vi "Dispose.vi"(8 "error in (no error)":errorcluster, 11 "ProductA":refnum<class "ProductA.lvclass">) -> (0 "error out":errorcluster)   [LabVIEW 2020, in "FactoryMethod.lvlib" / "FactoryMethodLazyEvaluation.lvlib" / "ProductA.lvclass"]
uses:
  ProductA.lvclass
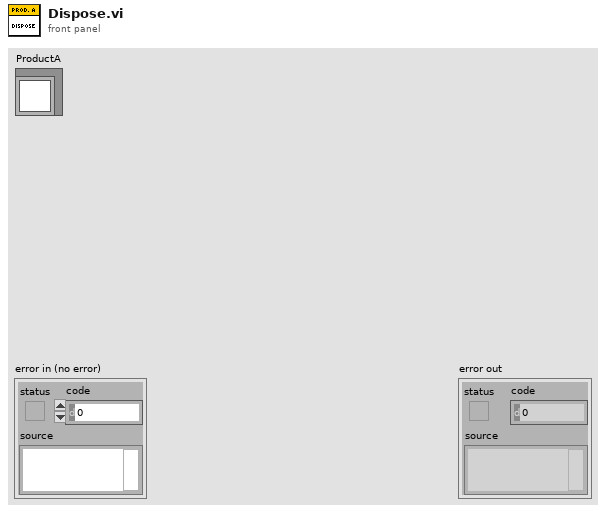
[diagram p1: front panel]
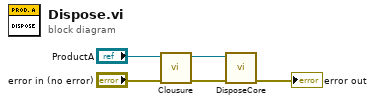
[diagram p0: block diagram]
diagram:
  n1 = call-dynamic "Clousure.vi"("error in (no error)"="error in (no error)", "ProductA"="ProductA") -> ("error out"=w3:errorcluster, "ProductA"=w1:refnum<class "ProductA.lvclass">)  [unwired: 8 in]
  n2 = call-dynamic "DisposeCore.vi"("error in (no error)"=w3, "ProductA"=w1) -> ("error out"=→"error out":errorcluster)  [unwired: 8 in, 1 out]
